vi "TML-clusters.vi"(7 "RS232-axis":u8=1 format="%0d", 8 "error in (no error)":errorcluster, 9 "value":dbl=22414.0, 10 "command":string="end", 11 "axis":u8=3) -> (0 "error out":errorcluster={"status"=TRUE, "code"=0, "source"="unknown TML command"}, 1 "expect return":T1(ring), 2 "command byte array":u8[](array[numeric]) format="%02x")   [LabVIEW 2011]
panel:
  in  "Known commands":T2(array[cluster])=[{"command name"="upd", "Parameter"=enum."none", "CommandArray"=[1, 8], "return"=FALSE}, {"command name"="cpa", "Parameter"=enum."none", "CommandArray"=[89, 9, 255, 255, 32, 0], "return"=FALSE}, {"command name"="mode pp3", "Parameter"=enum."none", "CommandArray"=[89, 9, 191, 193, 135, 1], "return"=FALSE}, {"command name"="endinit", "Parameter"=enum."none", "CommandArray"=[0, 32], "return"=FALSE}, {"command name"="axison", "Parameter"=enum."none", "CommandArray"=[1, 2], "return"=FALSE}, {"command name"="axisoff", "Parameter"=enum."none", "CommandArray"=[0, 2], "return"=FALSE}, {"command name"="mode sp", "Parameter"=enum."none", "CommandArray"=[89, 9, 187, 193, 131, 1], "return"=FALSE}, {"command name"="sap", "Parameter"=enum."I32", "CommandArray"=[132, 0], "return"=FALSE}, {"command name"="stop", "Parameter"=enum."none", "CommandArray"=[1, 196], "return"=FALSE}, {"command name"="reset", "Parameter"=enum."none", "CommandArray"=[4, 2], "return"=FALSE}, {"command name"="goto cal", "Parameter"=enum."none", "CommandArray"=[118, 0, 3, 178], "return"=FALSE}, {"command name"="goto abs", "Parameter"=enum."none", "CommandArray"=[118, 0, 3, 180], "return"=FALSE}, {"command name"="goto rel", "Parameter"=enum."none", "CommandArray"=[118, 0, 3, 181], "return"=FALSE}, {"command name"="goto range", "Parameter"=enum."none", "CommandArray"=[118, 0, 3, 179], "return"=FALSE}, {"command name"="readspi", "Parameter"=enum."I16", "CommandArray"=[176, 8, 0, 17], "return"=TRUE}, {"command name"="write16spi@32b+", "Parameter"=enum."I16", "CommandArray"=[144, 40, 3, 43], "return"=FALSE}, {"command name"="write32spi@32b+", "Parameter"=enum."I32", "CommandArray"=[144, 41, 3, 43], "return"=FALSE}, {"command name"="goto @var", "Parameter"=enum."I16", "CommandArray"=[118, 0], "return"=FALSE}, {"command name"="faultr", "Parameter"=enum."none", "CommandArray"=[28, 4], "return"=FALSE}, {"command name"="ping", "Parameter"=enum."none", "CommandArray"=[214, 0, 0, 17, 48, 0], "return"=TRUE}, {"command name"="eneeprom", "Parameter"=enum."none", "CommandArray"=[149, 0], "return"=FALSE}, {"command name"="end", "Parameter"=enum."none", "CommandArray"=[0, 1], "return"=FALSE}] {"CommandArray" format="%02x"}
  # "rev 2020 no old till vektors any more!"
  # "ping not tested, multiple returns?"
  # "90A8 ist (VAR16D), TypeMem = value16, SPI"
  # "76 01 ist call VAR16, needs return"
  # "was ist 9600?"
  # "format unknown to: @0xFFFF, only 16bit!"
  # "?blabla_x02b3"
  # "blax02b3="
  # "wie wäre es mit\n16x1234=\n32x1234="
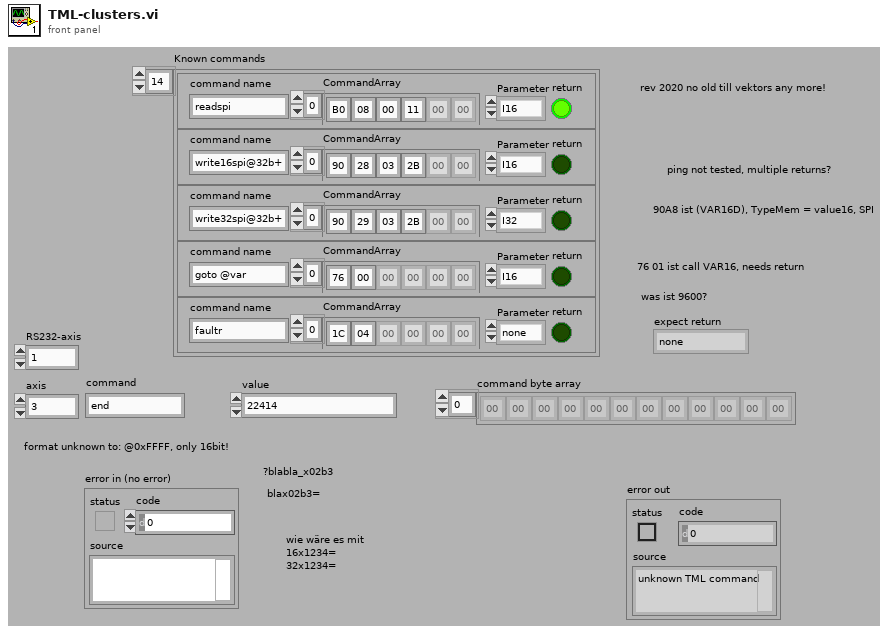
[diagram p1: front panel]
types:
  T1 = enum8{"none", "program32", "program16", "data32", "data16", "eprom32", "eprom16", "somethingelse32", "somethingelse16"}
  T2 = cluster{"command name":string, "Parameter":enum16{"none", "I16", "I32", "FixedI16.I16", "3Words"}, "CommandArray":u8[], "return":bool}[]
  T3 = enum16{"unknown", "i16", "u16", "i32", "u32", "fix32"}
  T4 = cluster{string[], u32[], enum16{"unknown", "i16", "u16", "i32", "u32", "fix32"}[], "comment":string[]}
  T5 = enum16{"unknown", "i16", "u16", "i32", "u32", "fix32"}[]
  T6 = cluster{"command name":string, "Parameter":enum16{"none", "I16", "I32", "FixedI16.I16", "3Words"}, "CommandArray":u8[], "return":bool}
  T7 = enum16{"none", "I16", "I32", "FixedI16.I16", "3Words"}
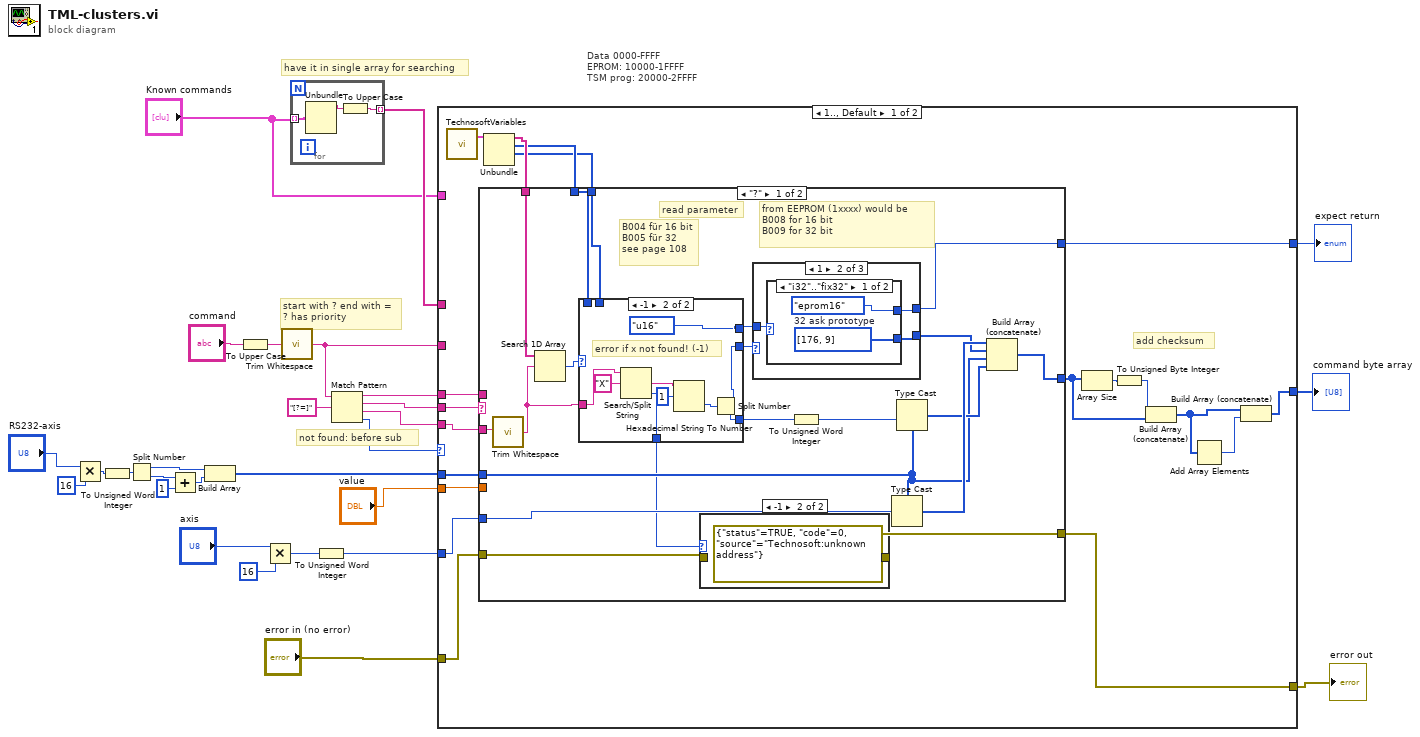
[diagram p0: block diagram]
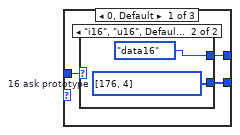
[diagram p3: hidden frame]
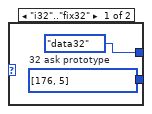
[diagram p4: hidden frame]
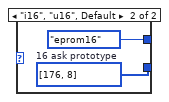
[diagram p5: hidden frame]
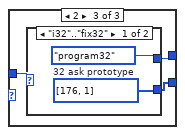
[diagram p6: hidden frame]
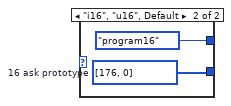
[diagram p7: hidden frame]
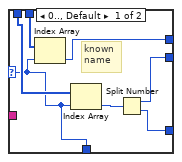
[diagram p8: hidden frame]
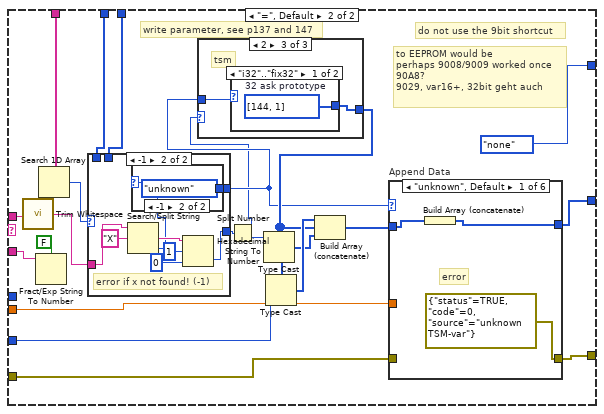
[diagram p9: hidden frame]
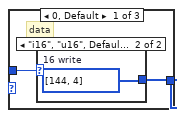
[diagram p10: hidden frame]
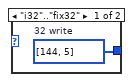
[diagram p11: hidden frame]
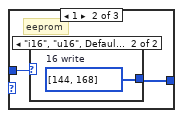
[diagram p12: hidden frame]
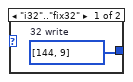
[diagram p13: hidden frame]
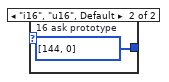
[diagram p14: hidden frame]
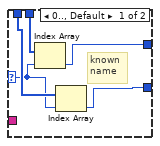
[diagram p15: hidden frame]
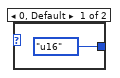
[diagram p16: hidden frame]
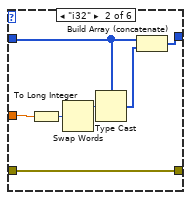
[diagram p17: hidden frame]
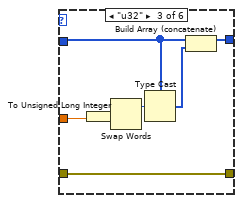
[diagram p18: hidden frame]
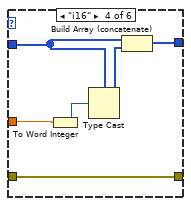
[diagram p19: hidden frame]
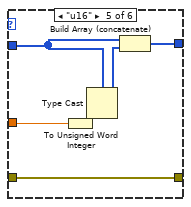
[diagram p20: hidden frame]
diagram:
  # "Data 0000-FFFF\nEPROM: 10000-1FFFF\nTSM prog: 20000-2FFFF"
  # "have it in single array for searching"
  # "not found: before sub"
  # "start with ? end with =\n? has priority"
  n1 = Multiply(x="RS232-axis", y=u16 16) -> (x*y=w13:u16)
  n2 = To Unsigned Word Integer(number=w13) -> (unsigned 16bit integer=w2:u16)
  n3 = Split Number(x=w2) -> (hi(x)=w12:u8, lo(x)=w11:u8)
  n4 = Add(x=w11, y=u8 1) -> (x+y=w10:u8)
  n5 = Build Array(w12, w10) -> (w5:u8[])
  n6 = To Upper Case(1:"command") -> (0:w4:string)
  n7 = Multiply(x="axis", y=u16 16) -> (x*y=w6:u16)
  n8 = call <vilib>:"Trim Whitespace.vi"("string"=w4) -> ("trimmed string"=w24:string)  [unwired: 1 in]
  n9 = for {
    tunnel: "Known commands" -> [w31] mode=indexing
    tunnel: [w29] -> w17 mode=indexing
    n10 = Unbundle(w31) -> ("command name"=w30:string)  [unwired: 3 out]
    n11 = To Upper Case(1:w30) -> (0:w29:string)
  }
  n12 = To Unsigned Word Integer(number=w6) -> (unsigned 16bit integer=w1:u16)
  n13 = Match Pattern(string=w24, regular expression="[?=]") -> (before substring=w21:string, match substring=w20:string, after substring=w19:string, offset past match=w22:i32)  [unwired: 1 out]
  n14 = case shown="1.., Default" w22 {
    tunnel: "error in (no error)" -> [w38 w211]
    tunnel: [w37 w210] -> w26
    tunnel: w24 -> [_ w209]
    tunnel: [w41 w208] -> w23
    tunnel: w21 -> [w49 _]
    tunnel: w20 -> [w50 _]
    tunnel: w19 -> [w48 _]
    tunnel: w1 -> [w47 w207]
    tunnel: "value" -> [w40 w206]
    tunnel: w17 -> [_ w205]
    tunnel: "Known commands" -> [_ w204]
    tunnel: w5 -> [w39 _]
    tunnel: [w32 w203] -> w3
    frame 1.., Default {
      # "add checksum"
      n15 = call "TechnosoftVariables.vi"() -> ("TSM variable table"=w35:T4)  [unwired: 1 in, 3 out]
      n16 = Unbundle(w35) -> (w36:string[], w34:u32[], w33:T5)  [unwired: 1 out]
      n17 = case shown="\"?\"" w50 {
        tunnel: w49 -> [_ w125]
        tunnel: w48 -> [w59 w120]
        tunnel: w36 -> [w70 w131]
        tunnel: w34 -> [w69 w118]
        tunnel: w47 -> [w68 w130]
        tunnel: [w64 w126] -> w44
        tunnel: w33 -> [w63 w117]
        tunnel: w40 -> [_ w128]
        tunnel: w39 -> [w60 _]
        tunnel: w38 -> [w52 w124]
        tunnel: [w51 w123] -> w37
        tunnel: [w54 T1."none" ("expect return")] -> w32
        frame "?" {
          # "from EEPROM (1xxxx) would be \nB008 for 16 bit\nB009 for 32 bit"
          # "read parameter"
          # "B004 für 16 bit\nB005 für 32\nsee page 108"
          n18 = call <vilib>:"Trim Whitespace.vi"("string"=w59) -> ("trimmed string"=w57:string)  [unwired: 1 in]
          n19 = Search 1D Array(1D array=w70, element=w57) -> (index of element=w58:i32)  [unwired: 1 out]
          n20 = case shown="-1" w58 {
            selector: w58 -> [w94 _]
            tunnel: w69 -> [w100 _]
            tunnel: [w96 w102] -> w66
            tunnel: w63 -> [w99 _]
            tunnel: [w98 T3."u16" ("type")] -> w62
            tunnel: w57 -> [_ w106]
            tunnel: [w95 w103] -> w55
            tunnel: [w94 w101] -> w53
            frame 0.., Default {
              # "known\nname"
              n21 = Index Array(array=w99, index=w94) -> (element=w98:T3)
              n22 = Index Array(array=w100, index=w94) -> (element=w97:u32)
              n23 = Split Number(x=w97) -> (hi(x)=w95:u16, lo(x)=w96:u16)
            }
            frame -1 {
              # "error if x not found! (-1)"
              n24 = Search/Split String(string=w106, search string/char (-)="X") -> (match + rest of string=w107:string, offset of match=w101:i32)  [unwired: 2 out]
              n25 = Hexadecimal String To Number(string=w107, offset=1) -> (number=w105:u32)  [unwired: 2 out]
              n26 = Split Number(x=w105) -> (hi(x)=w103:u16, lo(x)=w102:u16)
            }
          }
          n27 = case shown="-1" w53 {
            tunnel: w52 -> [w71 _]
            tunnel: [w71 errorcluster {"status"=TRUE, "code"=0, "source"="Technosoft:unknown address"} ("error in (no error)")] -> w51
            frame 0, Default {
            }
            frame -1 {
            }
          }
          n28 = case shown="1" w55 {
            tunnel: w62 -> [w75 w81 w88]
            tunnel: [w74 w82 w89] -> w61
            tunnel: [w73 w80 w87] -> w54
            frame 0, Default {
              n29 = case shown="\"i16\", \"u16\", Default" w75 {
                tunnel: [w77 w79] -> w74
                tunnel: [T1."data32" ("expect return") T1."data16" ("expect return")] -> w73
                frame "i32".."fix32" {
                  w77 = u8[] [176, 5]  # 32 ask prototype
                }
                frame "i16", "u16", Default {
                  w79 = u8[] [176, 4]  # 16 ask prototype
                }
              }
            }
            frame 1 {
              n30 = case shown="\"i32\"..\"fix32\"" w81 {
                tunnel: [w84 w86] -> w82
                tunnel: [T1."eprom16" ("expect return") T1."eprom16" ("expect return")] -> w80
                frame "i32".."fix32" {
                  w84 = u8[] [176, 9]  # 32 ask prototype
                }
                frame "i16", "u16", Default {
                  w86 = u8[] [176, 8]  # 16 ask prototype
                }
              }
            }
            frame 2 {
              n31 = case shown="\"i32\"..\"fix32\"" w88 {
                tunnel: [w91 w93] -> w89
                tunnel: [T1."program32" ("expect return") T1."program16" ("expect return")] -> w87
                frame "i32".."fix32" {
                  w91 = u8[] [176, 1]  # 32 ask prototype
                }
                frame "i16", "u16", Default {
                  w93 = u8[] [176, 0]  # 16 ask prototype
                }
              }
            }
          }
          n32 = To Unsigned Word Integer(number=w66) -> (unsigned 16bit integer=w56:u16)
          n33 = Type Cast(type=w60, x=w68) -> (*(type *) &x=w67:u8[])
          n34 = Type Cast(type=w60, x=w56) -> (*(type *) &x=w65:u8[])
          n35 = Build Array (concatenate)(w67, w61, w60, w65) -> (w64:u8[])
        }
        frame "=", Default {
          # "to EEPROM would be \nperhaps 9008/9009 worked once\n90A8?\n9029, var16+, 32bit geht auch"
          # "do not use the 9bit shortcut"
          # "write parameter, see p137 and 147"
          n36 = call <vilib>:"Trim Whitespace.vi"("string"=w125) -> ("trimmed string"=w114:string)  [unwired: 1 in]
          n37 = Fract/Exp String To Number(use system decimal point (T)=FALSE, string=w120) -> ()  [unwired: 4 out]
          n38 = Search 1D Array(1D array=w131, element=w114) -> (index of element=w115:i32)  [unwired: 1 out]
          n39 = case shown="-1" w115 {
            selector: w115 -> [w145 _]
            tunnel: w118 -> [w148 _]
            tunnel: [w144 w149] -> w113
            tunnel: w117 -> [w147 _]
            tunnel: [w146 w152] -> w116
            tunnel: w114 -> [_ w153]
            frame 0.., Default {
              # "known\nname"
              n40 = Index Array(array=w147, index=w145) -> (element=w146:T3)
              n41 = Index Array(array=w148, index=w145) -> (element=w144:u32)
            }
            frame -1 {
              # "error if x not found! (-1)"
              n42 = Search/Split String(string=w153, search string/char (-)="X") -> (match + rest of string=w154:string, offset of match=w150:i32)  [unwired: 2 out]
              n43 = case shown="-1" w150 {
                tunnel: [T3."u16" ("type") T3."unknown" ("type")] -> w152
                frame 0, Default {
                }
                frame -1 {
                }
              }
              n44 = Hexadecimal String To Number(string=w154, offset=1, default (0uL)=u32 0 ("default (0 U32)")) -> (number=w149:u32)  [unwired: 1 out]
            }
          }
          n45 = Split Number(x=w113) -> (hi(x)=w112:u16, lo(x)=w111:u16)
          n46 = case shown="2" w112 {
            tunnel: [w133 w136 w140] -> w121
            tunnel: w116 -> [w132 w137 w141]
            frame 0, Default {
              # "data"
              n47 = case shown="\"i16\", \"u16\", Default" w132 {
                tunnel: [w134 w135] -> w133
                frame "i32".."fix32" {
                  w134 = u8[] [144, 5]  # 32 write
                }
                frame "i16", "u16", Default {
                  w135 = u8[] [144, 4]  # 16 write
                }
              }
            }
            frame 1 {
              # "eeprom"
              n48 = case shown="\"i16\", \"u16\", Default" w137 {
                tunnel: [w138 w139] -> w136
                frame "i32".."fix32" {
                  w138 = u8[] [144, 9]  # 32 write
                }
                frame "i16", "u16", Default {
                  w139 = u8[] [144, 168]  # 16 write
                }
              }
            }
            frame 2 {
              # "tsm"
              n49 = case shown="\"i32\"..\"fix32\"" w141 {
                tunnel: [w142 w143] -> w140
                frame "i32".."fix32" {
                  w142 = u8[] [144, 1]  # 32 ask prototype
                }
                frame "i16", "u16", Default {
                  w143 = u8[] [144, 0]  # 16 ask prototype
                }
              }
            }
          }
          n50 = Type Cast(type=w121, x=w111) -> (*(type *) &x=w122:u8[])
          n51 = Type Cast(type=w121, x=w130) -> (*(type *) &x=w129:u8[])
          n52 = Build Array (concatenate)(w129, w121, w122) -> (w127:u8[])
          n53 = case "Append Data" shown="\"unknown\", Default" w116 {
            tunnel: w128 -> [_ w168 w175 w177 w183 w201]
            tunnel: w127 -> [w161 w166 w173 w181 w187 w191]
            tunnel: [w160 w165 w172 w179 w185 w202] -> w126
            tunnel: w124 -> [_ w162 w169 w176 w182 w188]
            tunnel: [errorcluster {"status"=TRUE, "code"=0, "source"="unknown TSM-var"} ("error in (no error)") w162 w169 w176 w182 w188] -> w123
            frame "unknown", Default {
              # "error"
              n54 = Build Array (concatenate)(w161) -> (w160:u8[])
            }
            frame "i32" {
              n55 = To Long Integer(number=w168) -> (32bit integer=w163:i32)
              n56 = Swap Words(1:w163) -> (0:w164:i32)
              n57 = Type Cast(type=w166, x=w164) -> (*(type *) &x=w167:u8[])
              n58 = Build Array (concatenate)(w166, w167) -> (w165:u8[])
            }
            frame "u32" {
              n59 = To Unsigned Long Integer(number=w175) -> (unsigned 32bit integer=w170:u32)
              n60 = Swap Words(1:w170) -> (0:w171:u32)
              n61 = Type Cast(type=w173, x=w171) -> (*(type *) &x=w174:u8[])
              n62 = Build Array (concatenate)(w173, w174) -> (w172:u8[])
            }
            frame "i16" {
              n63 = To Word Integer(number=w177) -> (16bit integer=w178:i16)
              n64 = Type Cast(type=w181, x=w178) -> (*(type *) &x=w180:u8[])
              n65 = Build Array (concatenate)(w181, w180) -> (w179:u8[])
            }
            frame "u16" {
              n66 = To Unsigned Word Integer(number=w183) -> (unsigned 16bit integer=w184:u16)
              n67 = Type Cast(type=w187, x=w184) -> (*(type *) &x=w186:u8[])
              n68 = Build Array (concatenate)(w187, w186) -> (w185:u8[])
            }
            frame "fix32" {
              n69 = Quotient & Remainder(x=w201, y=1.0) -> (x-y*floor(x/y)=w193:dbl, floor(x/y)=w199:dbl)
              n70 = Scale By Power Of 2(n=u16 16, x=u32 1) -> (x*2^n=w195:u32)
              n71 = Multiply(x=w195, y=w193) -> (x*y=w194:dbl)
              n72 = To Word Integer(number=w199) -> (16bit integer=w198:i16)
              n73 = To Unsigned Word Integer(number=w194) -> (unsigned 16bit integer=w192:u16)
              n74 = Type Cast(type=w191, x=w192) -> (*(type *) &x=w189:u8[])
              n75 = Type Cast(type=w191, x=w198) -> (*(type *) &x=w190:u8[])
              n76 = Build Array (concatenate)(w191, w189, w190) -> (w202:u8[])
            }
          }
        }
      }
      n77 = Array Size(array=w44) -> (size(s)=w46:i32)
      n78 = To Unsigned Byte Integer(number=w46) -> (unsigned 8bit integer=w45:u8)
      n79 = Build Array (concatenate)(w45, w44) -> (w43:u8[])
      n80 = Add Array Elements(numeric array=w43) -> (sum=w42:u8)
      n81 = Build Array (concatenate)(w43, w42) -> (w41:u8[])
    }
    frame -1 {
      # "command not a variable"
      n82 = Search 1D Array(1D array=w205, element=w209) -> (index of element=w212:i32)  [unwired: 1 out]
      n83 = case shown="0.." w212 {
        tunnel: w204 -> [_ w234]
        tunnel: w212 -> [_ w233]
        tunnel: [u8[] [] w224] -> w208
        tunnel: w211 -> [_ w222]
        tunnel: [errorcluster {"status"=TRUE, "code"=0, "source"="unknown TML command"} ("error in (no error)") w222] -> w210
        tunnel: w207 -> [_ w221]
        tunnel: w206 -> [_ w220]
        tunnel: [T1."none" ("expect return") w218] -> w203
        frame -1, Default {
          # "command not found"
        }
        frame 0.. {
          # "gibt nur \"readspi\""
          # "mindestens 1byte: 4F"
          # "expect return seems to be obsolete, always false, only with ?, would need RS232-axis"
          # "•  int    16-bit signed integer \n•  uint   16-bit unsigned integer \n•  fixed  32-bit fixed-point data with the 16MSB for the integer part and the 16LSB \n    for the factionary part.  \n•  long   32-bit signed integer \n•  ulong  32-bit unsigned integer"
          n84 = Index Array(array=w234, index=w233) -> (element=w232:T6)
          n85 = Unbundle(w232) -> ("Parameter"=w223:T7, "CommandArray"=w230:u8[], "return"=w219:bool)  [unwired: 1 out]
          n86 = Type Cast(type=w230, x=w221) -> (*(type *) &x=w231:u8[])
          n87 = case shown="\"I16\"" w223 {
            tunnel: w231 -> [w237 w244 w250 w265]
            tunnel: w220 -> [_ w243 w245 w263]
            tunnel: w230 -> [w236 w241 w249 w253]
            tunnel: [w235 w240 w247 w264] -> w228
            frame "none", Default {
              n88 = Build Array (concatenate)(w237, w236) -> (w235:u8[])
            }
            frame "I32" {
              n89 = To Long Integer(number=w243) -> (32bit integer=w238:i32)
              n90 = Swap Words(1:w238) -> (0:w239:i32)
              n91 = Type Cast(type=w241, x=w239) -> (*(type *) &x=w242:u8[])
              n92 = Build Array (concatenate)(w244, w241, w242) -> (w240:u8[])
            }
            frame "I16" {
              n93 = To Word Integer(number=w245) -> (16bit integer=w246:i16)
              n94 = Type Cast(type=w249, x=w246) -> (*(type *) &x=w248:u8[])
              n95 = Build Array (concatenate)(w250, w249, w248) -> (w247:u8[])
            }
            frame "FixedI16.I16" {
              n96 = Quotient & Remainder(x=w263, y=1.0) -> (x-y*floor(x/y)=w255:dbl, floor(x/y)=w261:dbl)
              n97 = Scale By Power Of 2(n=u16 16, x=u32 1) -> (x*2^n=w257:u32)
              n98 = Multiply(x=w257, y=w255) -> (x*y=w256:dbl)
              n99 = To Word Integer(number=w261) -> (16bit integer=w260:i16)
              n100 = To Unsigned Word Integer(number=w256) -> (unsigned 16bit integer=w254:u16)
              n101 = Type Cast(type=w253, x=w254) -> (*(type *) &x=w251:u8[])
              n102 = Type Cast(type=w253, x=w260) -> (*(type *) &x=w252:u8[])
              n103 = Build Array (concatenate)(w265, w253, w251, w252) -> (w264:u8[])
            }
          }
          n104 = Array Size(array=w228) -> (size(s)=w229:i32)
          n105 = To Unsigned Byte Integer(number=w229) -> (unsigned 8bit integer=w227:u8)
          n106 = Select(t=T1."somethingelse16" ("expect return"), s=w219, f=T1."none" ("expect return")) -> (s? t:f=w218:T1)
          n107 = Build Array (concatenate)(w227, w228) -> (w226:u8[])
          n108 = Add Array Elements(numeric array=w226) -> (sum=w225:u8)
          n109 = Build Array (concatenate)(w226, w225) -> (w224:u8[])
        }
      }
    }
  }
  "error out" <- w26
  "command byte array" <- w23
  "expect return" <- w3
